vi "string2array.vi"(11 "String":string="20160324081453,250.02,0.1205,0.000000,2.15,6.000,8.12,5.1,6.15,4.78021") -> (3 "array":dbl[](array[numeric]))   [LabVIEW 2015]
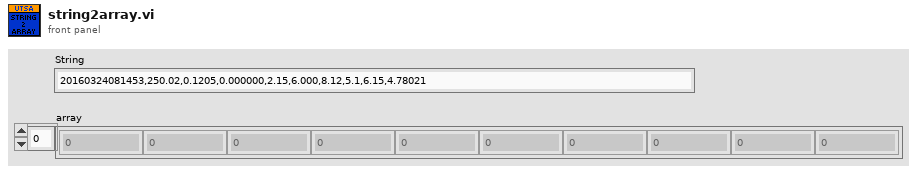
[diagram p1: front panel]
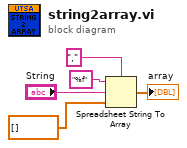
[diagram p0: block diagram]
diagram:
  n1 = Spreadsheet String To Array(delimiter (Tab)=",", format string="%f", spreadsheet string="String", array type (2D Dbl)=dbl[] []) -> (array=→"array":dbl[])
